vi "Hide Control.vi"(8 "error in (no error)":errorcluster, 11 "Ctrl Reference's in":refnum<class "Ctrl Reference's.lvclass">) -> (0 "error out":errorcluster, 3 "Ctrl Reference's out":refnum<class "Ctrl Reference's.lvclass">)   [LabVIEW 2023, in "Ctrl Reference's.lvclass"]
uses:
  Ctrl Reference's.lvclass
  Ctrl Reference's.lvclass/Ctrl Reference's.ctl
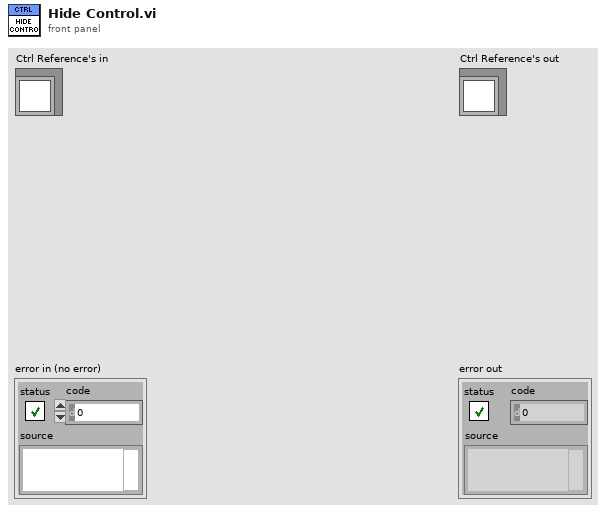
[diagram p1: front panel]
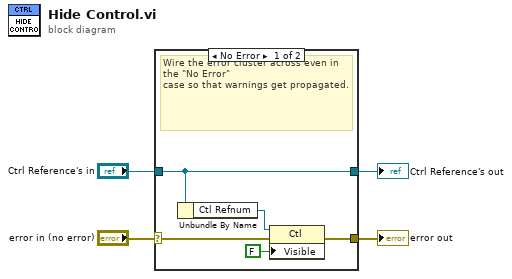
[diagram p0: block diagram]
diagram:
  n1 = case shown="No Error" "error in (no error)" {
    selector: "error in (no error)" -> [w7 w11]
    tunnel: [w5 w11] -> w3
    tunnel: [w9 w10] -> w1
    tunnel: "Ctrl Reference's in" -> [w9 w10]
    frame No Error {
      # "Wire the error cluster across even in the \"No Error\"\ncase so that warnings get propagated."
      n2 = Unbundle By Name(w9) -> ("Ctl Refnum"=w8:refnum<vi>)
      n3 = property class="Ctl"(reference=w8, error in=w7, "Visible"=FALSE) -> (error out=w5:errorcluster)  [unwired: 1 out]
    }
    frame Error {
    }
  }
  "error out" <- w3
  "Ctrl Reference's out" <- w1
